vi "ShotInterception_Init.vi"(0 "object in":refnum<class "ShotInterception.lvclass">, 5 "error in (no error)":errorcluster) -> (14 "object out":refnum<class "ShotInterception.lvclass">, 19 "error out":errorcluster)   [LabVIEW 2023, in "ShotInterception.lvclass"]
uses:
  ShotInterception.lvclass
  C:/Users/ebert/Documents/codes/SSL/repo/SSL_AI/NewSTP/Criteria/Criterion_class/Criterion.lvclass
  ShotInterception.lvclass/ShotInterception.ctl
  Criterion_class/Criterion.lvclass
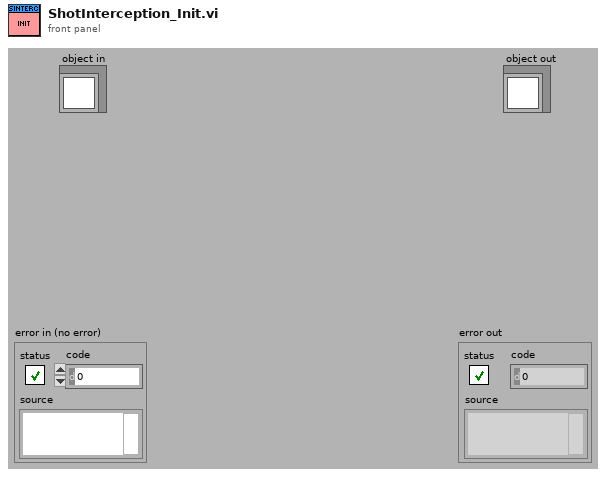
[diagram p1: front panel]
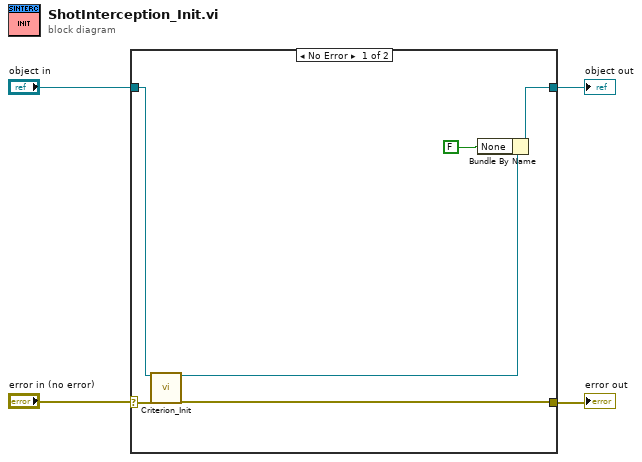
[diagram p0: block diagram]
diagram:
  n1 = case shown="No Error" "error in (no error)" {
    selector: "error in (no error)" -> [w7 w11]
    tunnel: "object in" -> [w8 w12]
    tunnel: [w10 w12] -> w3
    tunnel: [w5 w11] -> w1
    frame No Error {
      n2 = call "Criterion_Init.vi"("object in"=w8, "error in (no error)"=w7) -> ("object out"=w6:refnum<class "ShotInterception.lvclass">, "error out"=w5:errorcluster)  [unwired: 16 in]
      n3 = Bundle By Name(cluster=w6, "None"=FALSE) -> (w10:refnum<class "ShotInterception.lvclass">)
    }
    frame Error {
    }
  }
  "object out" <- w3
  "error out" <- w1
